vi "EXECUTION_CORE.vi"(8 "error in (no error)":errorcluster, 11 "Execution in":refnum<data-value>) -> (0 "error out":errorcluster, 3 "Execution out":refnum<data-value>)   [LabVIEW 2015, in "Execution.lvclass"]
uses:
  Execution.lvclass
  EXECUTION_STATUS.ctl
  Step.lvclass
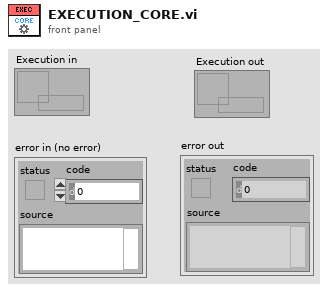
[diagram p1: front panel]
types:
  T1 = typedef "Execution.lvclass/EXECUTION_STATUS.ctl" = enum16{"Initializing ", "Disable", "Ready", "Running", "Finished"}
  T2 = typedef "Execution.lvclass/EXECUTION_CTRL_QUEUE_DATA.ctl" = cluster{"Msg":T3, "Data":variant}
  T3 = typedef "Execution.lvclass/EXECUTION_CTRL_MSG.ctl" = enum16{"EXECUTION_START", "EXECUTION_END", "EXECUTION_LOOP", "APPLICATION_STOP"}
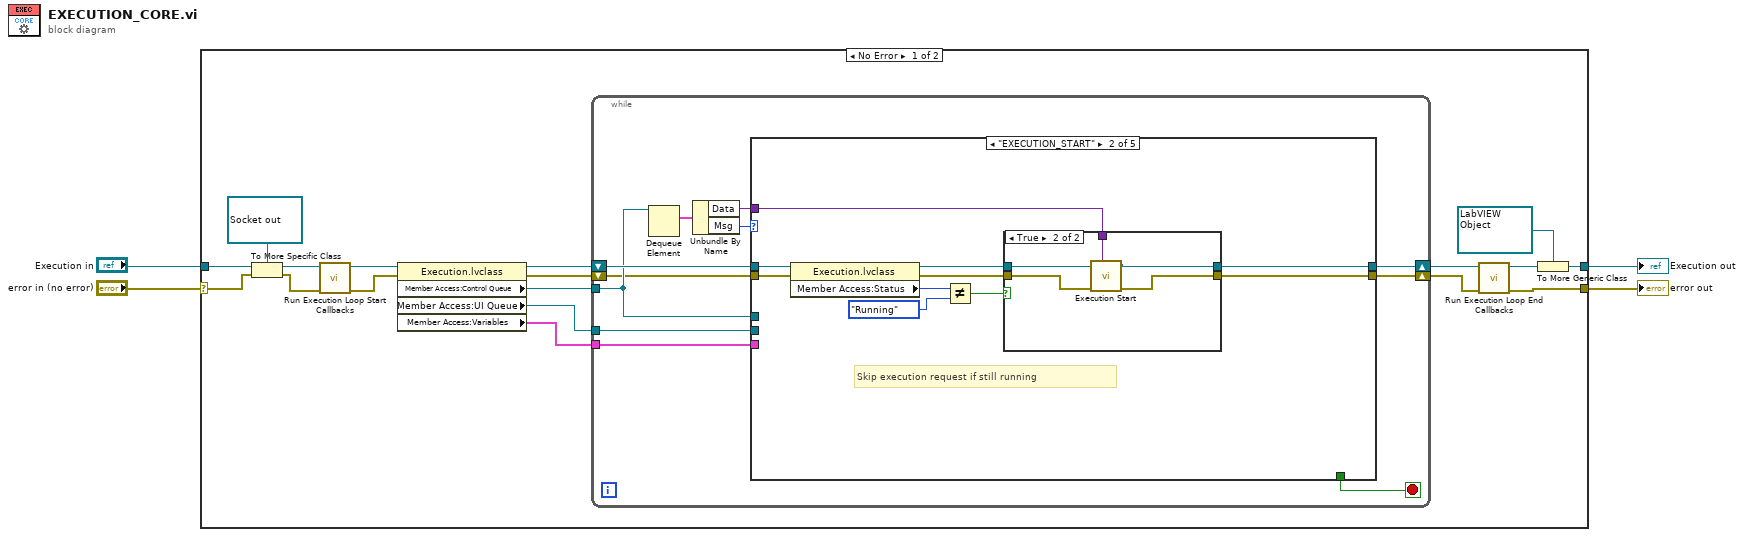
[diagram p0: block diagram]
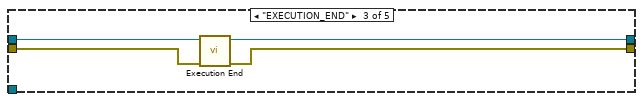
[diagram p4: hidden frame]
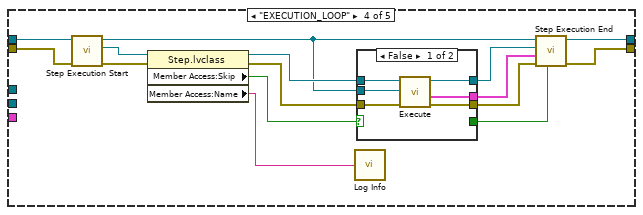
[diagram p5: hidden frame]
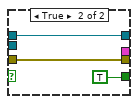
[diagram p6: hidden frame]
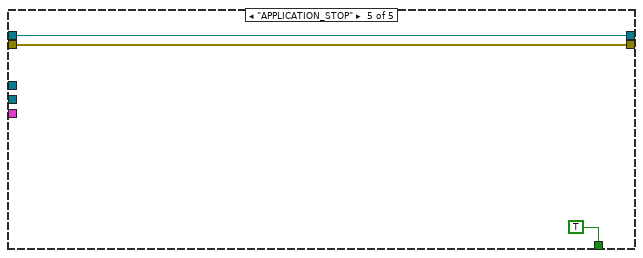
[diagram p7: hidden frame]
diagram:
  n1 = case shown="No Error" "error in (no error)" {
    selector: "error in (no error)" -> [w19 w85]
    tunnel: [w5 w85] -> w3
    tunnel: "Execution in" -> [w16 w84]
    tunnel: [w14 w84] -> w1
    frame No Error {
      n2 = To More Specific Class(target class=refnum<data-value> refnum ("reference out"), reference=w16, error in=w19) -> (specific class reference=w12:refnum<data-value>, error out=w11:errorcluster)
      n3 = call "Run Execution Loop Start Callbacks.vi"("error in (no error)"=w11, "Execution in"=w12) -> ("error out"=w7:errorcluster, "Execution out"=w8:refnum<data-value>)  [unwired: 8 in]
      n4 = property class="Execution.lvclass"(reference=w8, error in=w7) -> (reference out=w20:refnum<data-value>, error out=w18:errorcluster, "Member Access:Control Queue"=w21:refnum<queue>, "Member Access:UI Queue"=w17:refnum<queue>, "Member Access:Variables"=w13:cluster{"Name":string, "Value":variant}[])
      n5 = while {
        tunnel: w21 -> [w27]
        shift-right: [w30] -> w9
        shift-left: w18 -> [w26]
        tunnel: w17 -> [w28]
        shift-right: [w25] -> w10
        shift-left: w20 -> [w31]
        tunnel: w13 -> [w24]
        stop <- w29 stop-if-true
        n6 = Dequeue Element(queue=w27) -> (element=w33:T2)  [unwired: 2 in, 3 out]
        n7 = Unbundle By Name(w33) -> ("Data"=w23:variant, "Msg"=w32:T3)
        n8 = case shown="\"EXECUTION_START\"" w32 {
          tunnel: w31 -> [w34 w42 w56 w70 w81]
          tunnel: [w35 w44 w53 w68 w82] -> w30
          tunnel: [_ _ _ _ TRUE] -> w29
          tunnel: w28 -> [_ _ _ _ _]
          tunnel: w27 -> [_ _ _ _ _]
          tunnel: w26 -> [w35 w40 w54 w71 w82]
          tunnel: [w34 w45 w55 w63 w81] -> w25
          tunnel: w24 -> [_ _ _ _ _]
          tunnel: w23 -> [_ w43 _ _ _]
          frame Default {
          }
          frame "EXECUTION_START" {
            # "Skip execution request if still running"
            n9 = property class="Execution.lvclass"(reference=w42, error in=w40) -> (reference out=w41:refnum<data-value>, error out=w37:errorcluster, "Member Access:Status"=w39:T1)
            n10 = Not Equal?(x=w39, y=EXECUTION_STATUS."Running") -> (x != y?=w36:bool)
            n11 = case shown="True" w36 {
              tunnel: [w47 w52] -> w45
              tunnel: [w46 w51] -> w44
              tunnel: w43 -> [_ w50]
              tunnel: w41 -> [w47 w49]
              tunnel: w37 -> [w46 w48]
              frame False {
              }
              frame True {
                n12 = call "Execution Start.vi"("Execution Data"=w50, "error in (no error)"=w48, "Execution in"=w49) -> ("error out"=w51:errorcluster, "Execution out"=w52:refnum<data-value>)  [unwired: 7 in]
              }
            }
          }
          frame "EXECUTION_END" {
            n13 = call "Execution End.vi"("error in (no error)"=w54, "Execution in"=w56) -> ("error out"=w53:errorcluster, "Execution out"=w55:refnum<data-value>)  [unwired: 8 in]
          }
          frame "EXECUTION_LOOP" {
            n14 = call "Step Execution Start.vi"("error in (no error)"=w71, "Execution in"=w70) -> ("error out"=w67:errorcluster, "Step"=w61:refnum<class "Step.lvclass">, "Execution out"=w58:refnum<data-value>)  [unwired: 7 in]
            n15 = property class="Step.lvclass"(reference=w61, error in=w67) -> (reference out=w66:refnum<class "Step.lvclass">, error out=w65:errorcluster, "Member Access:Skip"=w64:bool, "Member Access:Name"=w57:string)
            n16 = call "Log Info.vi"("Message"=w57) -> ()  [unwired: 4 in, 1 out]
            n17 = case shown="False" w64 {
              tunnel: [w77 w79] -> w69
              tunnel: [w76 w80] -> w62
              tunnel: w66 -> [w75 w80]
              tunnel: w65 -> [w74 w79]
              tunnel: [w73 _] -> w60
              tunnel: [_ TRUE] -> w59
              tunnel: w58 -> [w72 _]
              frame False {
                n18 = call-dynamic "Execute.vi"("error in (no error)"=w74, "Execution"=w72, "StepBase in"=w75) -> ("error out"=w77:errorcluster, "Output Values"=w73:cluster{"Name":string, "Variant Data":variant}[], "StepBase out"=w76:refnum<class "Step.lvclass">)  [unwired: 6 in]
              }
              frame True {
              }
            }
            n19 = call "Step Execution End.vi"("Skipped"=w59, "error in (no error)"=w69, "Output Values"=w60, "Step"=w62, "Execution in"=w58) -> ("error out"=w68:errorcluster, "Execution out"=w63:refnum<data-value>)  [unwired: 5 in]
          }
          frame "APPLICATION_STOP" {
          }
        }
      }
      n20 = call "Run Execution Loop End Callbacks.vi"("error in (no error)"=w9, "Execution in"=w10) -> ("error out"=w5:errorcluster, "Execution out"=w6:refnum<data-value>)  [unwired: 8 in]
      n21 = To More Generic Class(target class=refnum<data-value> refnum ("Execution in"), reference=w6) -> (generic class reference=w14:refnum<data-value>)
    }
    frame Error {
    }
  }
  "error out" <- w3
  "Execution out" <- w1
